vi "Drive.vi"(1 "Turn":dbl, 2 "Forward":dbl) -> ()   [LabVIEW 2025]
uses:
  <vilib>/Rock Robotics/WPI/ThirdParty/REV Robotics/REVLib/Typedef/Spark MAX Control Type.ctl
  <vilib>/Rock Robotics/WPI/ThirdParty/navx-mxp/_TypeDefs/FRIC_navX_DeviceNumbersTypeDef.ctl
  <vilib>/Rock Robotics/Network Tables/NT Write Variant.vi
  <vilib>/Rock Robotics/Network Tables/NT Write Number.vi
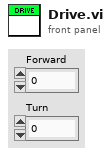
[diagram p1: front panel]
types:
  T1 = typedef "FRIC_navX_DeviceNumbersTypeDef.ctl" = enum16{"Dev0", "Dev1", "Dev2", "Dev3"}
  T2 = typedef "Spark MAX Control Type.ctl" = enum16{"Percent VBus", "Voltage", "Velocity", "Position", "Smart Motion", "Current", "Smart Velocity", "MAXMotion Position", "MAXMotion Velocity"}
  T3 = cluster{"Rollover":dbl, "Yaw":dbl, "Cont Yaw":dbl}
  T4 = typedef "WPI_MotorControlDeviceRef.ctl" = cluster{"DeviceStatus":errorcluster, "Type":T5, "PWM":cluster{"PWM Channel":T6, "DeadBand":T7}, "CAN":cluster{"Device Number":u8, "SetOutput VI Ref":variant, "GetOutput VI Ref":variant, "Enable VI Ref":variant, "Disable VI Ref":variant, "Data":variant}, "Invert":bool, "DIO PWM":cluster{"PWM \"Enable\" Channel":T6, "DIOChannel":T8, "PWM Rate":dbl}}
  T5 = typedef "WPI_MotorControlType.ctl" = enum16{"PWM", "CAN", "DIO PWM"}
  T6 = typedef "FPGA_DIOPWMChannel.ctl" = enum8{"PWM 0", "PWM 1", "PWM 2", "PWM 3", "PWM 4", "PWM 5", "PWM 6", "PWM 7", "PWM 8", "PWM 9", "PWM MXP 0", "PWM MXP 1", "PWM MXP 2", "PWM MXP 3", "PWM MXP 4", "PWM MXP 5", "PWM MXP 6", "PWM MXP 7", "PWM MXP 8", "PWM MXP 9", "Invalid"}
  T7 = typedef "WPI_PWMDeadband.ctl" = cluster{"Name":string, "maxPositivePwm":i32, "minPositivePwm":i32, "centerPwm":i32, "maxNegativePwm":i32, "minNegativePwm":i32, "angularRange":u16}
  T8 = typedef "FPGA_DIOChannel.ctl" = enum8{"DIO 0", "DIO 1", "DIO 2", "DIO 3", "DIO 4", "DIO 5", "DIO 6", "DIO 7", "DIO 8", "DIO 9", "DIO MXP 0", "DIO MXP 1", "DIO MXP 2", "DIO MXP 3", "DIO MXP 4", "DIO MXP 5", "DIO MXP 6", "DIO MXP 7", "DIO MXP 8", "DIO MXP 9", "DIO MXP 10", "DIO MXP 11", "DIO MXP 12", "DIO MXP 13", "DIO MXP 14", "DIO MXP 15", "SPI Port CS1", "SPI Port CS2", "SPI Port CS3", "SPI Port MISO", "SPI Port MOSI", "Invalid"}
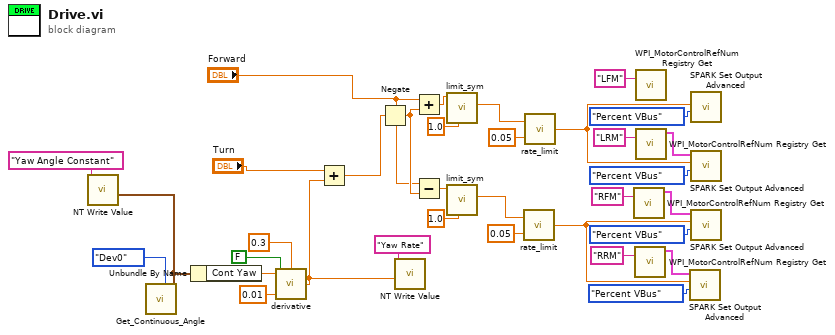
[diagram p0: block diagram]
diagram:
  n1 = call <vilib>:"Get_Continuous_Angle.vi"("Device Number"=FRIC_navX_DeviceNumbersTypeDef."Dev0") -> ("Continuous Angle"=w9:T3)  [unwired: 10 in]
  n2 = call-poly <vilib>:"NT Write Value.vi"("variant"=w9, "name"="Yaw Angle Constant") -> ()  [unwired: 9 in, 1 out]
  n3 = Unbundle By Name(w9) -> ("Cont Yaw"=w8:dbl)
  n4 = call "derivative.vi"("Time Constant"=0.3, "dt_ms"=0.01, "IC"=FALSE, "Input"=w8) -> ("Output"=w1:dbl)
  n5 = Add(x="Turn", y=w1) -> (x+y=w5:dbl)
  n6 = Negate(x=w5) -> (-x=w19:dbl)
  n7 = call-poly <vilib>:"NT Write Value.vi"("value"=w1, "name"="Yaw Rate") -> ()  [unwired: 9 in, 1 out]
  n8 = Add(x="Forward", y=w19) -> (x+y=w23:dbl)
  n9 = Subtract(x="Forward", y=w19) -> (x-y=w22:dbl)
  n10 = call "limit_sym.vi"("Limit"=1.0, "Input"=w23) -> ("Output"=w16:dbl)  [unwired: 9 in]
  n11 = call "limit_sym.vi"("Limit"=1.0, "Input"=w22) -> ("Output"=w14:dbl)  [unwired: 9 in]
  n12 = call "rate_limit.vi"("Rate Limit"=0.05, "In"=w14) -> ("Out"=w13:dbl)
  n13 = call "rate_limit.vi"("Rate Limit"=0.05, "In"=w16) -> ("Out"=w15:dbl)
  n14 = call <vilib>:"WPI_MotorControlRefNum Registry Get.vi"("refnum name"="RFM") -> ("MotorControlDevRef"=w31:T4)  [unwired: 9 in, 1 out]
  n15 = call <vilib>:"WPI_MotorControlRefNum Registry Get.vi"("refnum name"="RRM") -> ("MotorControlDevRef"=w28:T4)  [unwired: 9 in, 1 out]
  n16 = call <vilib>:"WPI_MotorControlRefNum Registry Get.vi"("refnum name"="LFM") -> ()  [unwired: 9 in, 2 out]
  n17 = call <vilib>:"WPI_MotorControlRefNum Registry Get.vi"("refnum name"="LRM") -> ("MotorControlDevRef"=w34:T4)  [unwired: 9 in, 1 out]
  n18 = call <vilib>:"SPARK Set Output Advanced.vi"("Control Mode"=Spark_MAX_Control_Type."Percent VBus", "Setpoint"=w13, "MotorControlDevRef"=w28) -> ()  [unwired: 7 in, 2 out]
  n19 = call <vilib>:"SPARK Set Output Advanced.vi"("Control Mode"=Spark_MAX_Control_Type."Percent VBus", "Setpoint"=w15) -> ()  [unwired: 8 in, 2 out]
  n20 = call <vilib>:"SPARK Set Output Advanced.vi"("Control Mode"=Spark_MAX_Control_Type."Percent VBus", "Setpoint"=w15, "MotorControlDevRef"=w34) -> ()  [unwired: 7 in, 2 out]
  n21 = call <vilib>:"SPARK Set Output Advanced.vi"("Control Mode"=Spark_MAX_Control_Type."Percent VBus", "Setpoint"=w13, "MotorControlDevRef"=w31) -> ()  [unwired: 7 in, 2 out]
